vi "Find Address Match.vi"(4 "error in (no error)":errorcluster, 6 "Misc Info":i32=-1, 7 "VISA resource name":refnum<visa-resource-name>) -> (0 "error out":errorcluster, 1 "Firmware":string, 2 "Matched Instrument":T1={"VISA Address"="", "Status"=0, "Manufacturer"="", "Model"="", "Info"="", "Info 2"="\n", "Misc Data"=variant} {"Status" format="%.0x"}, 3 "Model":string)   [LabVIEW 2024]
uses:
  Sub Controls/Instrument IDN.ctl
  SetupGlobals.vi
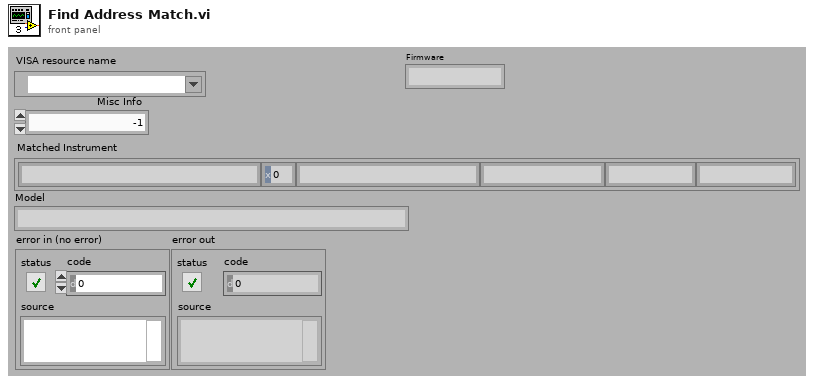
[diagram p1: front panel]
types:
  T1 = typedef "Instrument IDN.ctl" = cluster{"VISA Address":string, "Status":u16, "Manufacturer":string, "Model":string, "Info":string, "Info 2":string, "Misc Data":variant}
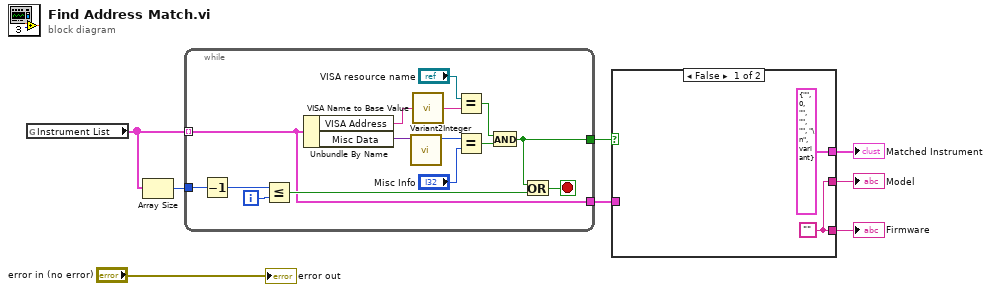
[diagram p0: block diagram]
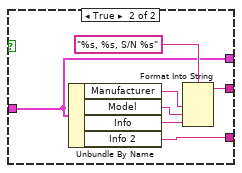
[diagram p2: hidden frame]
diagram:
  n1 = global read "SetupGlobals.vi" "Instrument List"() -> (w8:T1[])
  n2 = Array Size(array=w8) -> (size(s)=w7:i32)
  n3 = while {
    tunnel: w8 -> [w15] mode=indexing
    tunnel: w7 -> [w21]
    tunnel: [w13] -> w3
    tunnel: [w15] -> w4
    i -> [w20]
    stop <- w17 stop-if-true
    n4 = Decrement(x=w21) -> (x-1=w19:i32)
    n5 = Less Or Equal?(x=w19, y=w20) -> (x <= y?=w18:bool)
    n6 = Unbundle By Name(w15) -> ("VISA Address"=w23:string, "Misc Data"=w10:variant)
    n7 = call "Variant2Integer.vi"("Variant"=w10) -> ("data"=w11:i32)  [unwired: 9 in, 1 out]
    n8 = call "VISA Name to Base Value.vi"("String"=w23) -> ("String 2"=w14:string)
    n9 = Equal?(x="VISA resource name", y=w14) -> (x = y?=w16:bool)
    n10 = Equal?(x=w11, y="Misc Info") -> (x = y?=w12:bool)
    n11 = And(x=w16, y=w12) -> (x .and. y?=w13:bool)
    n12 = Or(x=w13, y=w18) -> (x .or. y?=w17:bool)
  }
  n13 = case shown="False" w3 {
    tunnel: [w24 w29] -> w5
    tunnel: [T1 {"VISA Address"="", "Status"=0, "Manufacturer"="", "Model"="", "Info"="", "Info 2"="\n", "Misc Data"=variant} ("f") w27] -> w6
    tunnel: w4 -> [_ w27]
    tunnel: [w24 w26] -> w1
    frame False {
      w24 = ""
    }
    frame True {
      n14 = Unbundle By Name(w27) -> ("Manufacturer"=w30:string, "Model"=w31:string, "Info"=w32:string, "Info 2"=w26:string)
      n15 = Format Into String(format string="%s, %s, S/N %s", w30, w31, w32) -> (resulting string=w29:string)  [unwired: 2 in, 1 out]
    }
  }
  "Matched Instrument" <- w6
  "Model" <- w5
  "Firmware" <- w1
  "error out" <- "error in (no error)"
